vi "Read Patch Header.vi"(8 "Index":u32, 11 "Patch DATA IN":u8[](array[numeric])) -> (0 "Index+8":u32, 1 "PatchHeader":T1, 3 "Patch DATA OUT":u8[](array[numeric]))   [LabVIEW 2017]
uses:
  PatchHeader.ctl
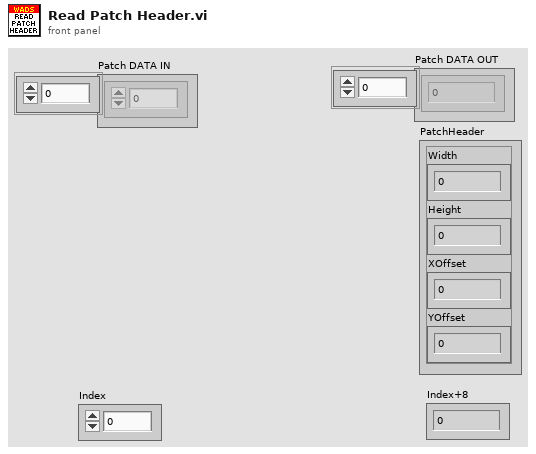
[diagram p1: front panel]
types:
  T1 = typedef "PatchHeader.ctl" = cluster{"Width":u16, "Height":u16, "XOffset":i16, "YOffset":i16}
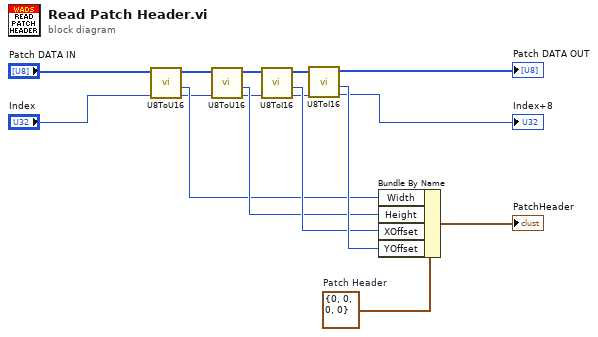
[diagram p0: block diagram]
diagram:
  w11 = T1 {"Width"=0, "Height"=0, "XOffset"=0, "YOffset"=0}  # Patch Header
  n1 = call "U8ToU16.vi"("Index"="Index", "Input U8 Array"="Patch DATA IN") -> ("Index+2"=w5:u32, "Output U16"=w12:u16, "Output U8 Array"=w6:u8[])  [unwired: 3 in]
  n2 = call "U8ToU16.vi"("Index"=w5, "Input U8 Array"=w6) -> ("Index+2"=w8:u32, "Output U16"=w13:u16, "Output U8 Array"=w7:u8[])  [unwired: 3 in]
  n3 = call "U8ToI16.vi"("Index"=w8, "Input U8 Array"=w7) -> ("Index+2"=w9:u32, "Output I16"=w14:i16, "Output U8 Array"=w10:u8[])  [unwired: 3 in]
  n4 = call "U8ToI16.vi"("Index"=w9, "Input U8 Array"=w10) -> ("Index+2"=→"Index+8":u32, "Output I16"=w15:i16, "Output U8 Array"=→"Patch DATA OUT":u8[])  [unwired: 3 in]
  n5 = Bundle By Name(cluster=w11, "Width"=w12, "Height"=w13, "XOffset"=w14, "YOffset"=w15) -> (→"PatchHeader":T1)
